vi "Ex3.vi"() -> ()   [LabVIEW 2015]
uses:
  <vilib>/rvi/Emulation/niFpgaGetClockAttributes.vi
  <vilib>/rvi/Emulation/niFpgaSctlEmulationGetInTimedLoop.vi
  <vilib>/rvi/Emulation/niFpgaEmulationReportErrorSimple.vi
  <vilib>/rvi/eio/common/nirviEmuTemplateMethod_errors.vi
  <vilib>/rvi/Emulation/niFpgaCriticalErrorInLSC.vi
  <vilib>/eio/EIONode/EIONode.xnode
panel:
  out "Waveform Chart":i16(graph)
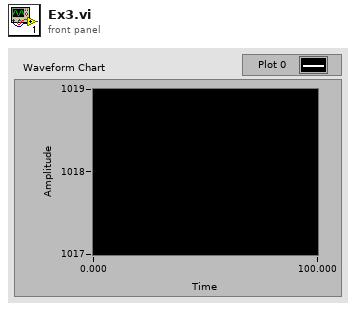
[diagram p1: front panel]
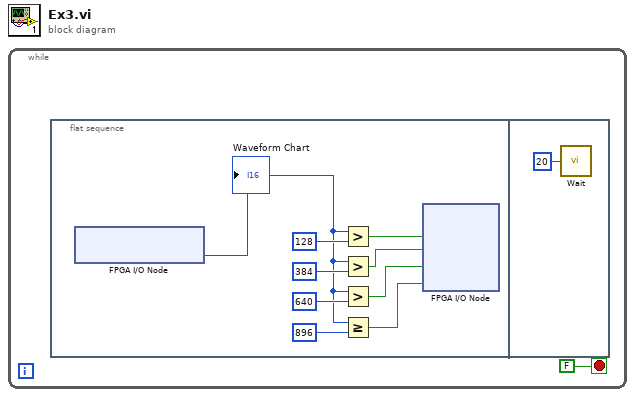
[diagram p0: block diagram]
diagram:
  n1 = while {
    stop <- FALSE stop-if-true
    n2 = flat-sequence {
      frame #0 {
        n3 = xnode "FPGA I/O Node"() -> ("ConnectorC/AI0"=w2:i16)  [unwired: 1 in, 1 out]
        "Waveform Chart" <- w2
        n4 = Greater?(x=w2, y=128) -> (0:w7:bool)
        n5 = Greater?(x=w2, y=384) -> (0:w6:bool)
        n6 = Greater?(x=w2, y=640) -> (0:w5:bool)
        n7 = Greater Or Equal?(x=w2, y=896) -> (x >= y?=w3:bool)
        n8 = xnode "FPGA I/O Node"("LED0"=w7, "LED1"=w6, "LED2"=w5, "LED3"=w3) -> ()  [unwired: 4 in, 4 out]
      }
      frame #1 {
        n9 = call "Wait"("Count(Ticks)"=u32 20) -> ()  [unwired: 1 out]
      }
    }
  }
